vi "Panel Data Entry.vi"() -> (0 "Run 2":i32=1, 1 "Unit Number 2":string="DGnn", 2 "Device Description 2":string="GE HEWH 1", 3 "Chamber Setting 2":string="58,50", 5 "Test Type 2":string="HEWH-MAN_OV")   [LabVIEW 2009]
panel:
  in  "Complete":bool
  in  "Unit Number":string="DGnn"
  in  "Chamber Setting":string="58,50"
  in  "Run":i32=1
  in  "Device Description":string="GE HEWH 1"
  in  "Test Type":string="HEWH-MAN_OV"
  # "Enter Test Data"
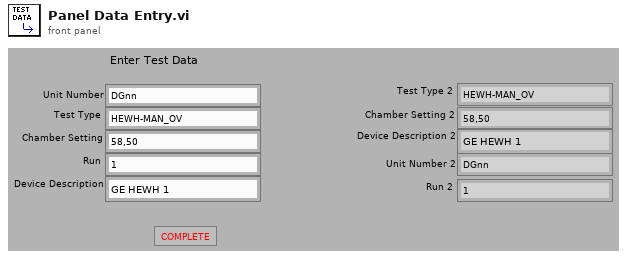
[diagram p1: front panel]
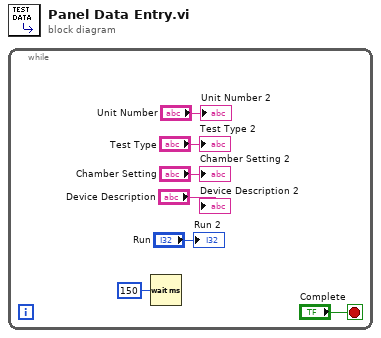
[diagram p0: block diagram]
diagram:
  n1 = while {
    stop <- "Complete" stop-if-true
    n2 = Wait (ms)(milliseconds to wait=u32 150) -> ()  [unwired: 1 out]
    "Unit Number 2" <- "Unit Number"
    "Test Type 2" <- "Test Type"
    "Chamber Setting 2" <- "Chamber Setting"
    "Device Description 2" <- "Device Description"
    "Run 2" <- "Run"
  }
